vi "Event Handler.vi"(8 "error in":errorcluster, 11 "Listbox in":refnum<class "Multi Column Listbox.lvclass">) -> (0 "error out":errorcluster, 3 "Listbox out":refnum<class "Multi Column Listbox.lvclass">)   [LabVIEW 2013, in "Table Manager.lvlib" / "Multi Column Listbox.lvclass"]
uses:
  Multi Column Listbox.lvclass
  Multi Column Listbox.lvclass/Multi Column Listbox.ctl
  <vilib>/Utility/miscctls.llb/LVPositionTypeDef.ctl
  TagSelectModule/Source/editor node/tag select module editor node.lvclass
  Table Manager.lvlib
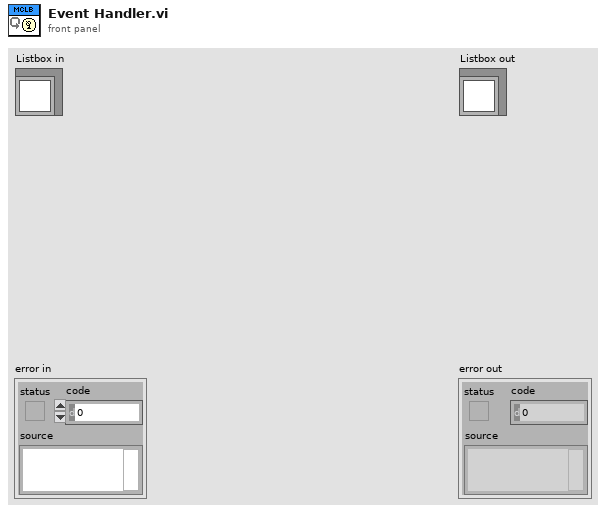
[diagram p1: front panel]
types:
  T1 = typedef "LVPositionTypeDef.ctl" = cluster{"Left":i32, "Top":i32}
  T2 = typedef "NISE_CEF_Node.lvclass/RefreshUIEvent.ctl" = refnum<user-event>
  T3 = typedef "tag select module editor node.lvclass/object ref.ctl" = cluster{"engine":refnum<data-value>, "Node Ref":refnum<data-value>}
  T4 = typedef "control module editor.lvclass/dialog output action.ctl" = enum16{"Tag Created", "Tag Selected", "Set Default", "disconnect"}
  T5 = typedef "LVRowAndColumnTypeDef.ctl" = cluster{"Row":i32, "Column":i32}
  T6 = typedef "LVPoint32TypeDef.ctl" = cluster{"Horizontal":i32, "Vertical":i32}
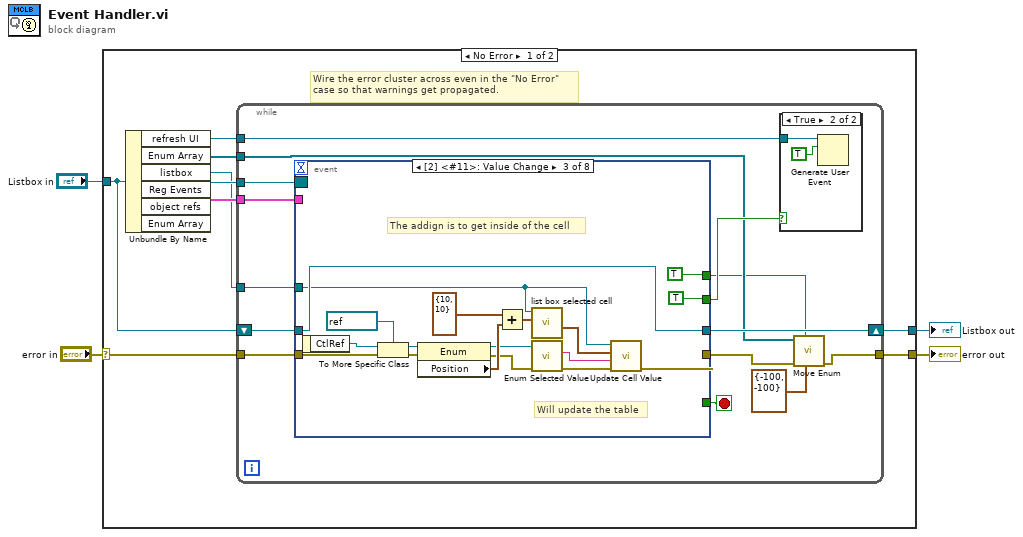
[diagram p0: block diagram]
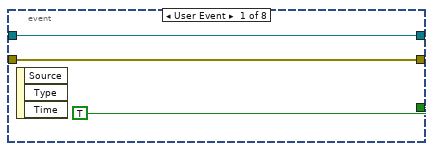
[diagram p3: hidden frame]
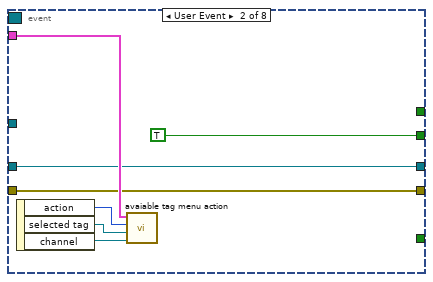
[diagram p4: hidden frame]
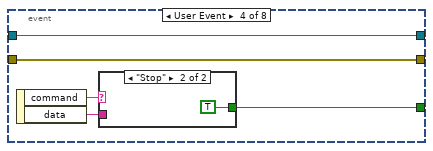
[diagram p5: hidden frame]
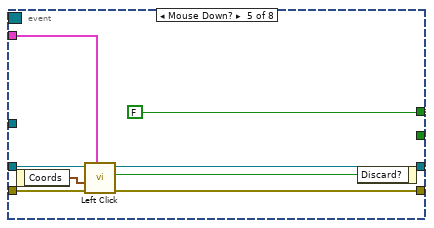
[diagram p7: hidden frame]
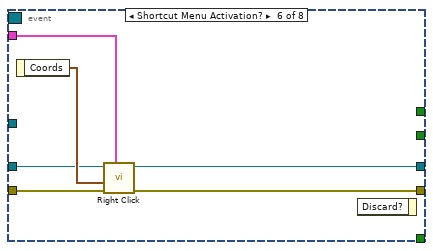
[diagram p8: hidden frame]
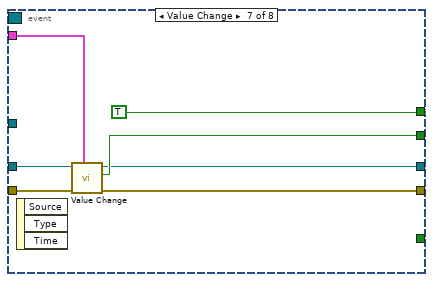
[diagram p9: hidden frame]
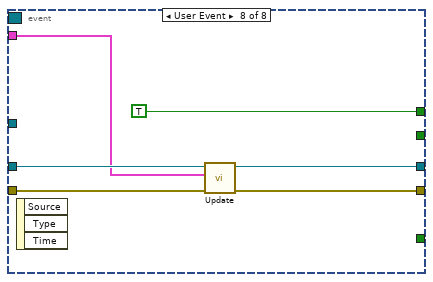
[diagram p10: hidden frame]
diagram:
  n1 = case shown="No Error" "error in" {
    selector: "error in" -> [w9 w92]
    tunnel: [w8 w92] -> w2
    tunnel: [w13 w91] -> w3
    tunnel: "Listbox in" -> [w12 w91]
    frame No Error {
      # "Wire the error cluster across even in the \"No Error\"\ncase so that warnings get propagated."
      n2 = Unbundle By Name(w12) -> ("refresh UI"=w6:T2, "Enum Array"=w5:refnum<vi>[], "listbox"=w7:refnum<vi>, "Reg Events"=w11:refnum<event-registration>, "object refs"=w10:T3)  [unwired: 1 out]
      n3 = while {
        shift-right: [w23] -> w13
        shift-left: w12 -> [w24]
        tunnel: w11 -> [w26]
        tunnel: w10 -> [w25]
        tunnel: w9 -> [w22]
        tunnel: [w18] -> w8
        tunnel: w5 -> [w20]
        tunnel: w7 -> [w17]
        tunnel: w6 -> [w16]
        stop <- w27 stop-if-true
        n4 = event shown="[2] <#11>: Value Change" {
          selector: w26 -> [_ _ _ _ _ _ _ _]
          dyn-events: _ -> [_ _ _ _ _ _ _ _]
          timeout: _ -> [_ _ _ _ _ _ _ _]
          tunnel: [TRUE _ _ w58 _ _ _ _] -> w27
          tunnel: w25 -> [_ w38 _ _ w70 w74 w80 w88]
          tunnel: w24 -> [w31 w37 w57 w62 w65 w76 w83 w90]
          tunnel: [w31 w37 w57 w62 w71 w75 w78 w89] -> w23
          tunnel: w22 -> [w30 w33 w46 w61 w68 w73 w82 w87]
          tunnel: [w30 w33 w44 w61 w67 w72 w81 w86] -> w19
          tunnel: [_ TRUE ("changed") TRUE ("changed") _ _ _ w79 _] -> w21
          tunnel: [_ _ TRUE _ FALSE _ TRUE TRUE] -> w14
          tunnel: w17 -> [_ _ w55 _ _ _ _ _]
          event User Event {
            n5 = event-data() -> ()  [unwired: 1 in, 3 out]
          }
          event User Event {
            n6 = event-data() -> ("action"=w39:T4, "selected tag"=w36:refnum<class "tag descriptor.lvclass">, "channel"=w35:refnum<class "TBM channel.lvclass">)  [unwired: 1 in]
            n7 = call "avaiable tag menu action.vi"("channel"=w35, "selected tag"=w36, "action"=w39, "object ref"=w38) -> ()  [unwired: 6 in, 2 out]
          }
          event Value Change {
            # "Will update the table"
            # "The addign is to get inside of the cell"
            n8 = event-data() -> ("CtlRef"=w56:refnum<vi>)  [unwired: 1 in]
            n9 = To More Specific Class(target class=refnum<vi> refnum ("Enum"), reference=w56, error in=w46) -> (specific class reference=w42:refnum<vi>, error out=w45:errorcluster)
            n10 = property class="Enum"(reference=w42, error in=w45) -> (reference out=w41:refnum<vi>, error out=w40:errorcluster, "Position"=w50:T1)
            n11 = Add(x=T1 {"Left"=10, "Top"=10} ("y"), y=w50) -> (x+y=w48:T1)
            n12 = call "list box selected cell.vi"("Coords"=w48, "MulticolumnListbox in"=w55) -> ("cell position"=w51:T5)  [unwired: 6 in, 3 out]
            n13 = call "Enum Selected Value.vi"("error in"=w40, "Enum"=w41) -> ("error out"=w43:errorcluster, "Value"=w47:string)  [unwired: 7 in, 1 out]
            n14 = call "Update Cell Value.vi"("error in"=w43, "Value"=w47, "cell position in"=w51, "MulticolumnListbox in"=w55) -> ("error out"=w44:errorcluster)  [unwired: 6 in, 1 out]
          }
          event User Event {
            n15 = event-data() -> ("command"=w60:string, "data"=w59:string)  [unwired: 1 in]
            n16 = case shown="\"Stop\"" w60 {
              tunnel: [_ TRUE] -> w58
              tunnel: w59 -> [_ _]
              frame Default {
              }
              frame "Stop" {
              }
            }
          }
          event Mouse Down? {
            n17 = event-data() -> ("Coords"=w69:T6)  [unwired: 1 in]
            n18 = call-dynamic "Left Click.vi"("object refs"=w70, "error in"=w68, "Coords"=w69, "Multi Column Listbox in"=w65) -> ("error out"=w67:errorcluster, "Discard?"=w66:bool, "Multi Column Listbox out"=w71:refnum<class "Multi Column Listbox.lvclass">)  [unwired: 5 in]
            n19 = event-data("Discard?"=w66) -> ()  [unwired: 1 in, 1 out]
          }
          event Shortcut Menu Activation? {
            n20 = event-data() -> ("Coords"=w77:T6)  [unwired: 1 in]
            n21 = call-dynamic "Right Click.vi"("object refs"=w74, "error in (no error)"=w73, "Coords"=w77, "Multi Column Listbox in"=w76) -> ("error out"=w72:errorcluster, "Multi Column Listbox out"=w75:refnum<class "Multi Column Listbox.lvclass">)  [unwired: 6 in]
            n22 = event-data() -> ()  [unwired: 2 in, 1 out]
          }
          event Value Change {
            n23 = event-data() -> ()  [unwired: 1 in, 3 out]
            n24 = call-dynamic "Value Change.vi"("objects"=w80, "error in"=w82, "Multi Column Listbox in"=w83) -> ("error out"=w81:errorcluster, "Update?"=w79:bool, "Multi Column Listbox out"=w78:refnum<class "Multi Column Listbox.lvclass">)  [unwired: 6 in]
          }
          event User Event {
            n25 = event-data() -> ()  [unwired: 1 in, 3 out]
            n26 = call-dynamic "Update.vi"("error in"=w87, "object ref in"=w88, "Multi Column Listbox in"=w90) -> ("error out"=w86:errorcluster, "Multi Column Listbox out"=w89:refnum<class "Multi Column Listbox.lvclass">)  [unwired: 6 in, 1 out]
          }
        }
        n27 = case shown="True" w21 {
          tunnel: w16 -> [_ w28]
          frame False {
          }
          frame True {
            n28 = Generate User Event(user event=w28, event data cluster=TRUE ("event data")) -> ()  [unwired: 2 in, 2 out]
          }
        }
        n29 = call "Move Enum.vi"("position"=T1 {"Left"=-100, "Top"=-100}, "move?"=w14, "error in"=w19, "Array"=w20) -> ("error out"=w18:errorcluster)  [unwired: 7 in]
      }
    }
    frame Error {
    }
  }
  "error out" <- w2
  "Listbox out" <- w3
